vi "ThermoCouple_Datafile_Create.vi"(8 "error in (no error)":errorcluster) -> (0 "error out":errorcluster, 3 "path out":path)   [LabVIEW 2022 SP3]
uses:
  <vilib>/Utility/file.llb/Write Delimited Spreadsheet (string).vi
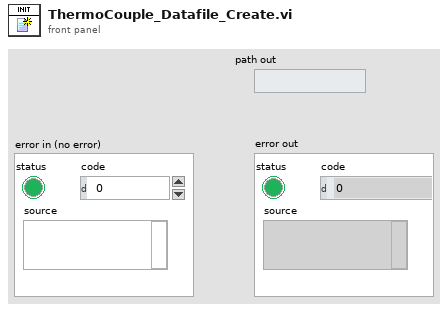
[diagram p1: front panel]
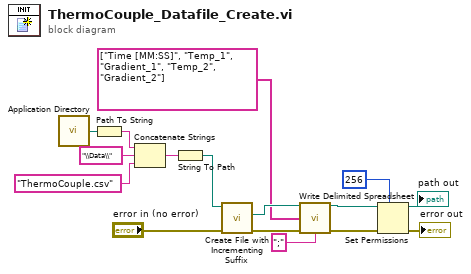
[diagram p0: block diagram]
diagram:
  n1 = call <vilib>:"Application Directory.vi"() -> ("Application Directory"=w13:path)
  n2 = Path To String(path=w13) -> (string=w14:string)
  n3 = Concatenate Strings(w14, "\\Data\\", "ThermoCouple.csv" ("string")) -> (w11:string)
  n4 = String To Path(string=w11) -> (path=w10:path)
  n5 = call <vilib>:"Create File with Incrementing Suffix.vi"("error in (no error)"="error in (no error)", "file path"=w10) -> ("error out"=w8:errorcluster, "actual path"=w3:path)  [unwired: 7 in, 1 out]
  n6 = call-poly <vilib>:"Write Delimited Spreadsheet.vi"("file path (dialog if empty)"=w3, "1D data"=string[] ["Time [MM:SS]", "Temp_1", "Gradient_1", "Temp_2", "Gradient_2"], "error in (no error)"=w8, "delimiter (\\t)"=";" ("delimiter (\\t)")) -> ("new file path (Not A Path if cancelled)"=w6:path, "error out"=w5:errorcluster)  [unwired: 10 in]
  n7 = Set Permissions(7:i16 256 ("permissions"), 8:w5, 11:w6) -> (0:→"error out":errorcluster, 3:→"path out":path)  [unwired: 2 in]
